vi "Enable Waveform.vi"(8 "error in (no error)":errorcluster, 9 "Enable Waveform (Disable)":bool, 10 "Channel (1:CH1)":u16(ring)=1 items=["CH1"=1, "CH2"=2], 11 "VISA resource name":refnum<visa-resource-name>) -> (0 "error out":errorcluster, 3 "VISA resource name out":refnum<visa-resource-name>)   [LabVIEW 2015, in "Siglent SPD3000 Series.lvlib"]
doc: "Controls the selected channel to show waveform or number.\n\n<B>Note:</B>\nThis VI is invalid for the SPD3303C models."
uses:
  <instrlib>/Siglent SPD3000 Series/Siglent SPD3000 Series.lvlib
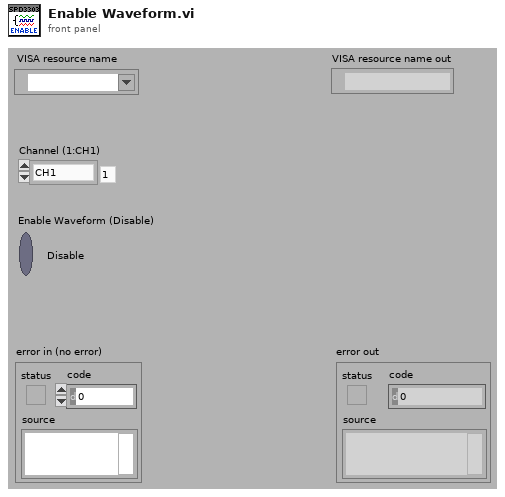
[diagram p1: front panel]
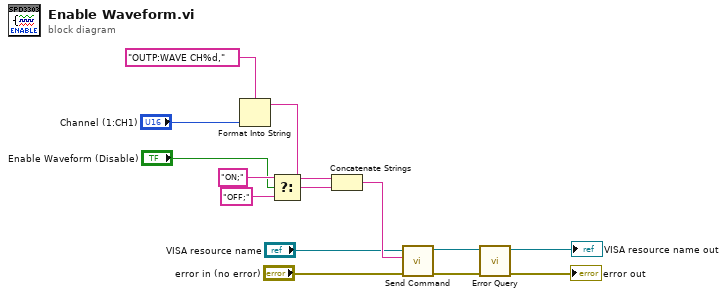
[diagram p0: block diagram]
diagram:
  n1 = Format Into String(format string="OUTP:WAVE CH%d," ("写入缓冲区"), "Channel (1:CH1)") -> (resulting string=w8:string)  [unwired: 2 in, 1 out]
  n2 = Select(t="ON;" ("写入缓冲区"), s="Enable Waveform (Disable)", f="OFF;" ("写入缓冲区")) -> (s? t:f=w9:string)
  n3 = Concatenate Strings(w8, w9) -> (w6:string)
  n4 = call <instrlib>:"Send Command.vi"("error in (no error)"="error in (no error)", "Write Buffer (\"\")"=w6, "VISA resource name"="VISA resource name") -> ("error out"=w13:errorcluster, "VISA resource name out"=w14:refnum<visa-resource-name>)  [unwired: 7 in]
  n5 = call <instrlib>:"Error Query.vi"("error in (no error)"=w13, "VISA resource name"=w14) -> ("error out"=→"error out":errorcluster, "VISA resource name out"=→"VISA resource name out":refnum<visa-resource-name>)  [unwired: 6 in, 2 out]
